vi "RegisterSettings.vi"(8 "error in":errorcluster, 11 "MainFGV_data":T1={"TestDir"=path "", "TestName"="", "task"="", "data_file"=refnum, "burts_file"=refnum, "log_file"=refnum, "AcqQueue"=refnum, "StartTime"=timestamp(0 s since 1904-01-01), "config_channels"=[], "DAQmx Device"="", "Advanced"={"rate"=1652.0, "duration"=1.0, "thr"=100.0, "preTrigger"=100.0, "cutoff"=-3.0, "Filtro"=enum."Desativado", "highPass"=1000.0, "lowPass"=1000.0, "updateTime"=50.0}, "running"=FALSE, "hammerIndex"=0} {"Advanced"."updateTime" format="%#_g ms"; "Advanced"."lowPass" format="%#_g Hz"; "Advanced"."highPass" format="%#_g Hz"; "Advanced"."cutoff" format="%#_g dB"; "Advanced"."preTrigger" format="%#_g ms"; "Advanced"."thr" format="%#_g N"; "Advanced"."duration" format="%#_g s"; "Advanced"."rate" min=1652.0 max=51200.0 format="%#_g Hz"}) -> (0 "error out":errorcluster, 3 "MainFGV_data out":T1={"TestDir"=path "", "TestName"="", "task"="", "data_file"=refnum, "burts_file"=refnum, "log_file"=refnum, "AcqQueue"=refnum, "StartTime"=timestamp(0 s since 1904-01-01), "config_channels"=[], "DAQmx Device"="", "Advanced"={"rate"=1652.0, "duration"=1.0, "thr"=100.0, "preTrigger"=100.0, "cutoff"=-3.0, "Filtro"=enum."Desativado", "highPass"=1000.0, "lowPass"=1000.0, "updateTime"=50.0}, "running"=FALSE, "hammerIndex"=0} {"Advanced"."updateTime" format="%#_g ms"; "Advanced"."lowPass" format="%#_g Hz"; "Advanced"."highPass" format="%#_g Hz"; "Advanced"."cutoff" format="%#_g dB"; "Advanced"."preTrigger" format="%#_g ms"; "Advanced"."thr" format="%#_g N"; "Advanced"."duration" format="%#_g s"; "Advanced"."rate" min=1652.0 max=51200.0 format="%#_g Hz"})   [LabVIEW 2016]
uses:
  MainFGV_data.ctl
  Settings/config_board.ctl
  Settings/Advanced/AdvancedConfig.ctl
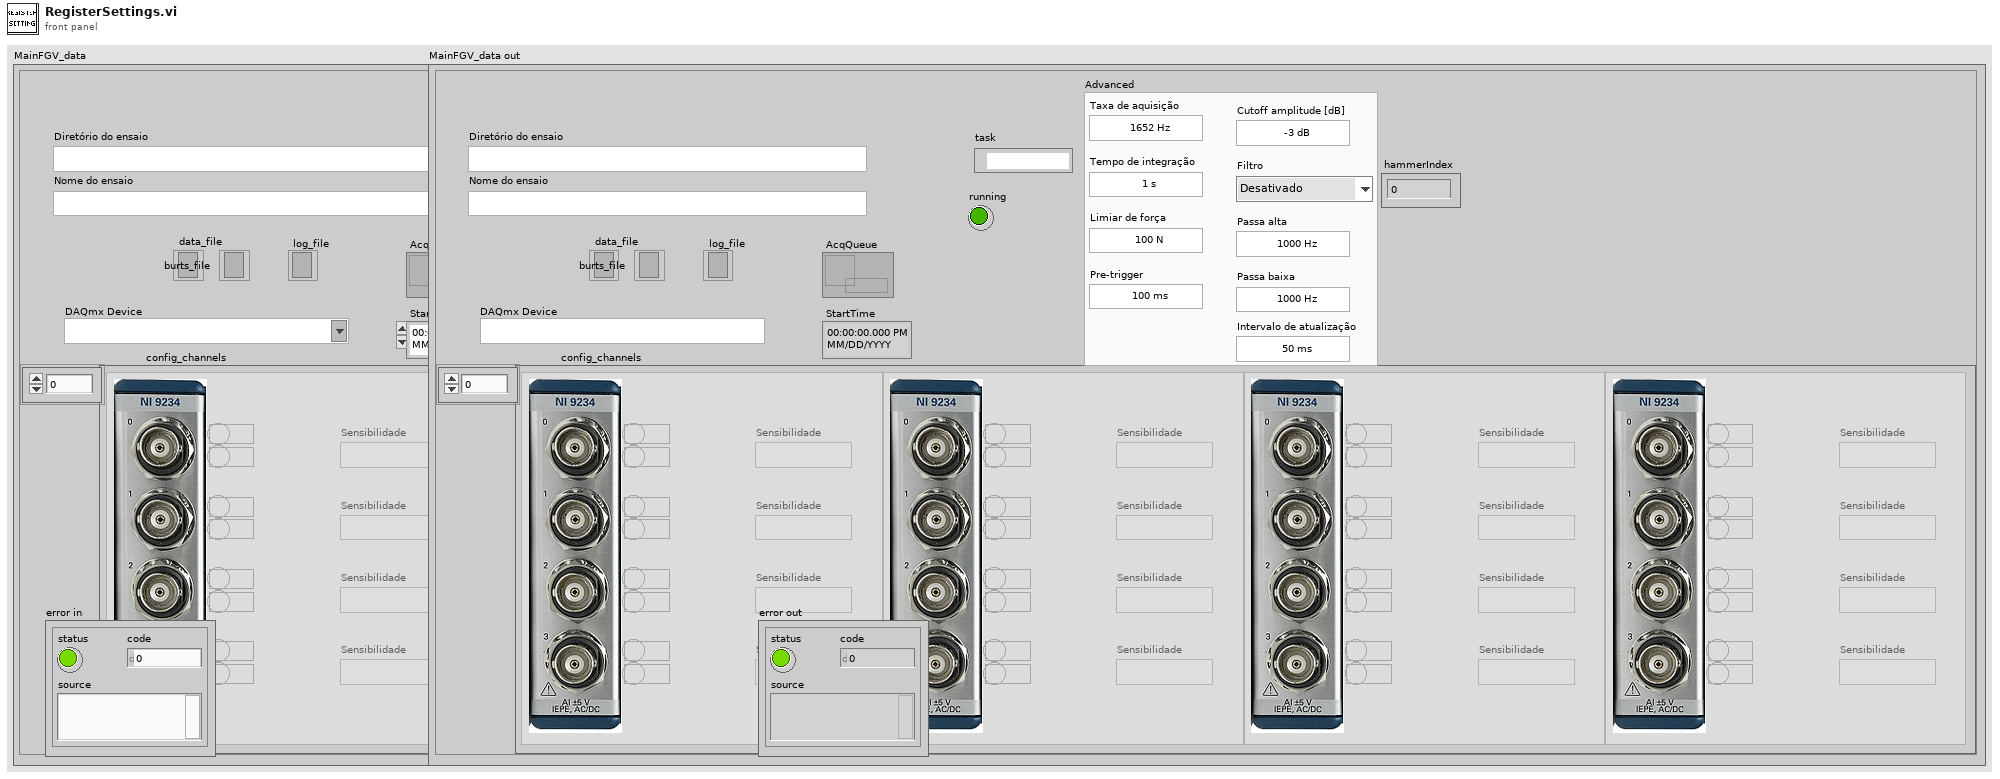
[diagram p1: front panel]
types:
  T1 = typedef "MainFGV_data.ctl" = cluster{"TestDir":path, "TestName":string, "task":refnum<k21>, "data_file":refnum<file>, "burts_file":refnum<file>, "log_file":refnum<file>, "AcqQueue":refnum<queue>, "StartTime":timestamp, "config_channels":T2[], "DAQmx Device":tag, "Advanced":T3, "running":bool, "hammerIndex":i32}
  T2 = typedef "config_board.ctl" = cluster{"Sens 1":dbl, "active 1":bool, "type 1":bool, "type 2":bool, "active 2":bool, "Sens 2":dbl, "type 3":bool, "active 3":bool, "Sens 3":dbl, "type 4":bool, "active 4":bool, "Sens 4":dbl}
  T3 = typedef "AdvancedConfig.ctl" = cluster{"rate":dbl, "duration":dbl, "thr":dbl, "preTrigger":dbl, "cutoff":dbl, "Filtro":enum16{"Desativado", "Passa banda", "Passa alta", "Passa baixa"}, "highPass":dbl, "lowPass":dbl, "updateTime":dbl}
  T4 = enum16{"open", "replace", "create", "open or create", "replace or create", "replace or create with confirmation"}
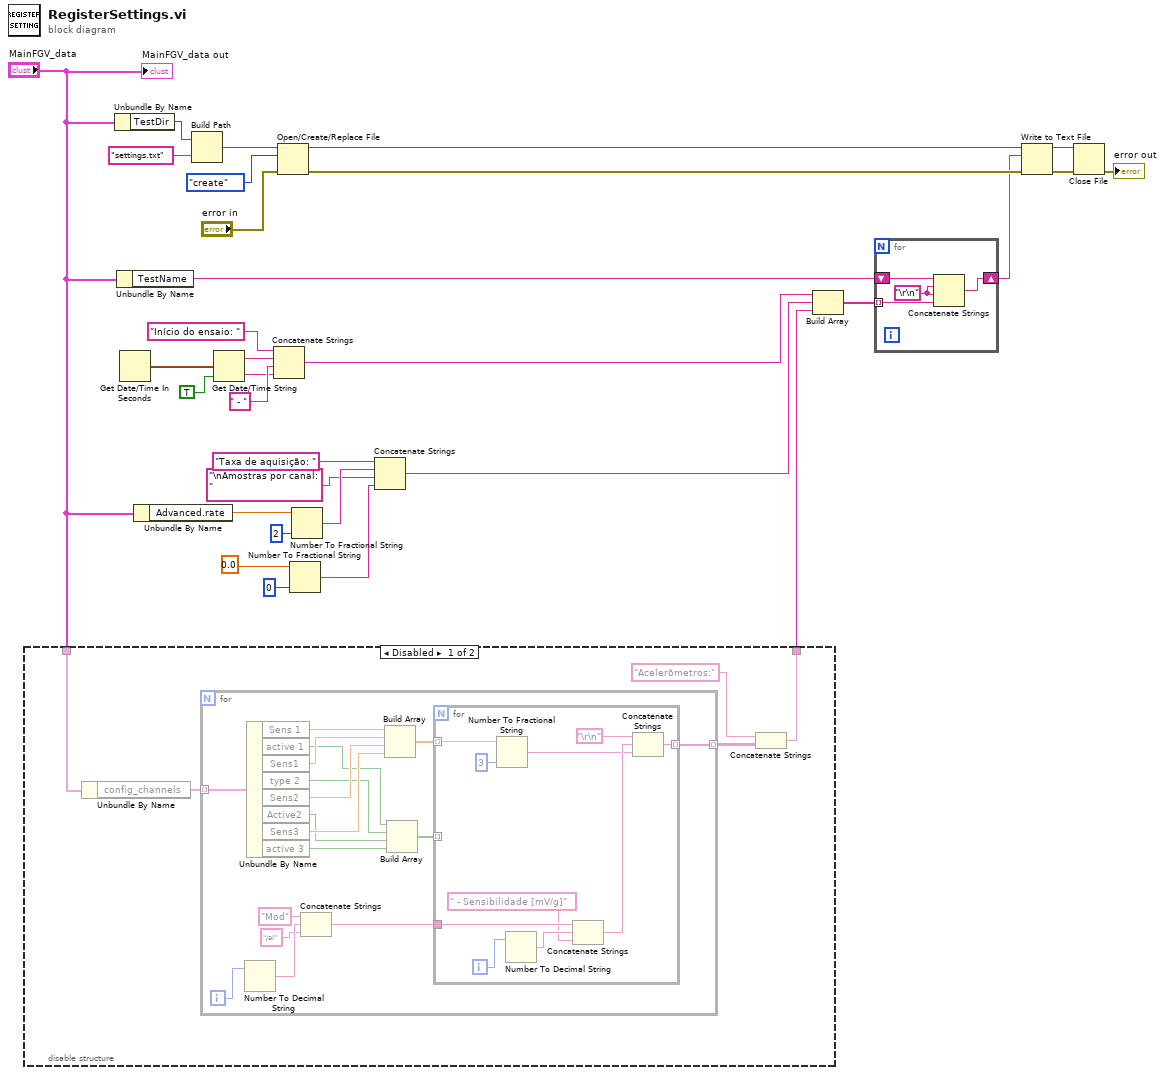
[diagram p0: block diagram]
diagram:
  n1 = disable-structure shown="Disabled" {
    disable-tunnel: "MainFGV_data" -> [w34 _]
    disable-tunnel: [w32 _] -> w12
    frame Disabled {
      n2 = Unbundle By Name(w34) -> ("config_channels"=w36:T2[])
      n3 = for {
        tunnel: w36 -> [w52] mode=indexing
        tunnel: [w37] -> w35 mode=indexing
        i -> [w53]
        n4 = Number To Decimal String(number=w53) -> (decimal integer string=w41:string)  [unwired: 1 in]
        n5 = Unbundle By Name(w52) -> ("Sens 1"=w51:dbl, "active 1"=w44:bool, "Sens1"=w50:dbl, "type 2"=w45:bool, "Sens2"=w49:dbl, "Active2"=w46:bool, "Sens3"=w48:dbl, "active 3"=w47:bool)
        n6 = Concatenate Strings("Mod" ("string"), w41, "/ai" ("string")) -> (w38:string)
        n7 = Build Array(w51, w50, w49, w48) -> (w42:dbl[])
        n8 = Build Array(w44, w45, w46, w47) -> (w43:bool[])
        n9 = for {
          tunnel: w43 -> [_] mode=indexing
          tunnel: w42 -> [w59] mode=indexing
          tunnel: w38 -> [w62]
          tunnel: [w54] -> w37 mode=indexing
          i -> [w63]
          n10 = Number To Fractional String(number=w59, precision (6)=i16 3) -> (F-format string=w56:string)  [unwired: 2 in]
          n11 = Number To Decimal String(number=w63) -> (decimal integer string=w61:string)  [unwired: 1 in]
          n12 = Concatenate Strings(w62, w61, " - Sensibilidade [mV/g]" ("string")) -> (w57:string)
          n13 = Concatenate Strings("\r\n", w57, w56) -> (w54:string)
        }
      }
      n14 = Concatenate Strings("Acelerômetros:" ("string"), w35) -> (w32:string)
    }
    frame Enabled {
    }
  }
  n15 = Unbundle By Name("MainFGV_data") -> ("TestDir"=w31:path)
  n16 = Unbundle By Name("MainFGV_data") -> ("TestName"=w3:string)
  n17 = Get Date/Time In Seconds() -> (seconds since 1Jan1904=w2:timestamp)
  n18 = Unbundle By Name("MainFGV_data") -> ("Advanced.rate"=w21:dbl)
  n19 = Build Path(base path=w31, name or relative path="settings.txt") -> (appended path=w29:path)
  n20 = Get Date/Time String(seconds (now)=w2, want seconds? (F)=TRUE) -> (date string=w24:string, time string=w23:string)  [unwired: 1 in]
  n21 = Concatenate Strings("Início do ensaio: " ("string"), w24, " - " ("string"), w23) -> (w14:string)
  n22 = Open/Create/Replace File(file path (use dialog)=w29, error in="error in", operation (0:open)=T4."create") -> (refnum out=w7:refnum<file>, error out=w9:errorcluster)  [unwired: 3 in, 1 out]
  n23 = Number To Fractional String(number=0.0, precision (6)=i16 0) -> (F-format string=w16:string)  [unwired: 2 in]
  n24 = Number To Fractional String(number=w21, precision (6)=i16 2) -> (F-format string=w19:string)  [unwired: 2 in]
  n25 = Concatenate Strings("Taxa de aquisição: " ("string"), w19, "\nAmostras por canal: " ("string"), w16) -> (w13:string)
  n26 = Build Array(w14, w13, w12) -> (w11:string[])
  n27 = for {
    tunnel: w11 -> [w66] mode=indexing
    shift-right: [w64] -> w8
    shift-left: w3 -> [w67]
    w65 = "\r\n"
    n28 = Concatenate Strings(w67, w65, w65, w66) -> (w64:string)
  }
  n29 = Write to Text File(file (use dialog)=w7, text=w8, error in=w9) -> (refnum out=w5:refnum<file>, error out=w6:errorcluster)  [unwired: 1 in, 1 out]
  n30 = Close File(refnum=w5, error in=w6) -> (error out=→"error out":errorcluster)  [unwired: 1 out]
  "MainFGV_data out" <- "MainFGV_data"
